vi "test4-MappingRelationshipByLocalRegistration.vi"(8 "error in (no error)":errorcluster, 11 "TestCase in":refnum<class "testcase-CSMStatusStateRegisterUnregister.lvclass">) -> (0 "error out":errorcluster, 3 "TestCase out":refnum<class "testcase-CSMStatusStateRegisterUnregister.lvclass">)   [LabVIEW 2017, in "testcase-CSMStatusStateRegisterUnregister.lvclass"]
uses:
  testcase-CSMStatusStateRegisterUnregister.lvclass
  <vilib>/addons/_JKI Toolkits/VI Tester/TestCase.llb/TestCase.lvclass
  src/user.lib/_NEVSTOP/Communicable State Machine(CSM)/Communicable State Machine.lvlib
  C:/Program Files (x86)/National Instruments/LabVIEW 2017/vi.lib/addons/_JKI Toolkits/VI Tester/TestCase.llb/TestCase.lvclass
panel:
  out "Entries After Removal":T1(array[cluster])
  out "Error Array 2":errorcluster[](array[cluster])
  out "Rules 3":T1(array[cluster])
  out "Status In Registry 3":string[](array[string])
  out "Rules 4":T1(array[cluster])
  out "Status In Registry 4":string[](array[string])
  out "Loop Count 2":i32
  out "Loop Count":i32
  out "Error Array":errorcluster[](array[cluster])
  out "Rules 2":T1(array[cluster])
  out "Status In Registry 2":string[](array[string])
  out "Status In Registry 1":string[](array[string])
  out "Rules 1":T1(array[cluster])
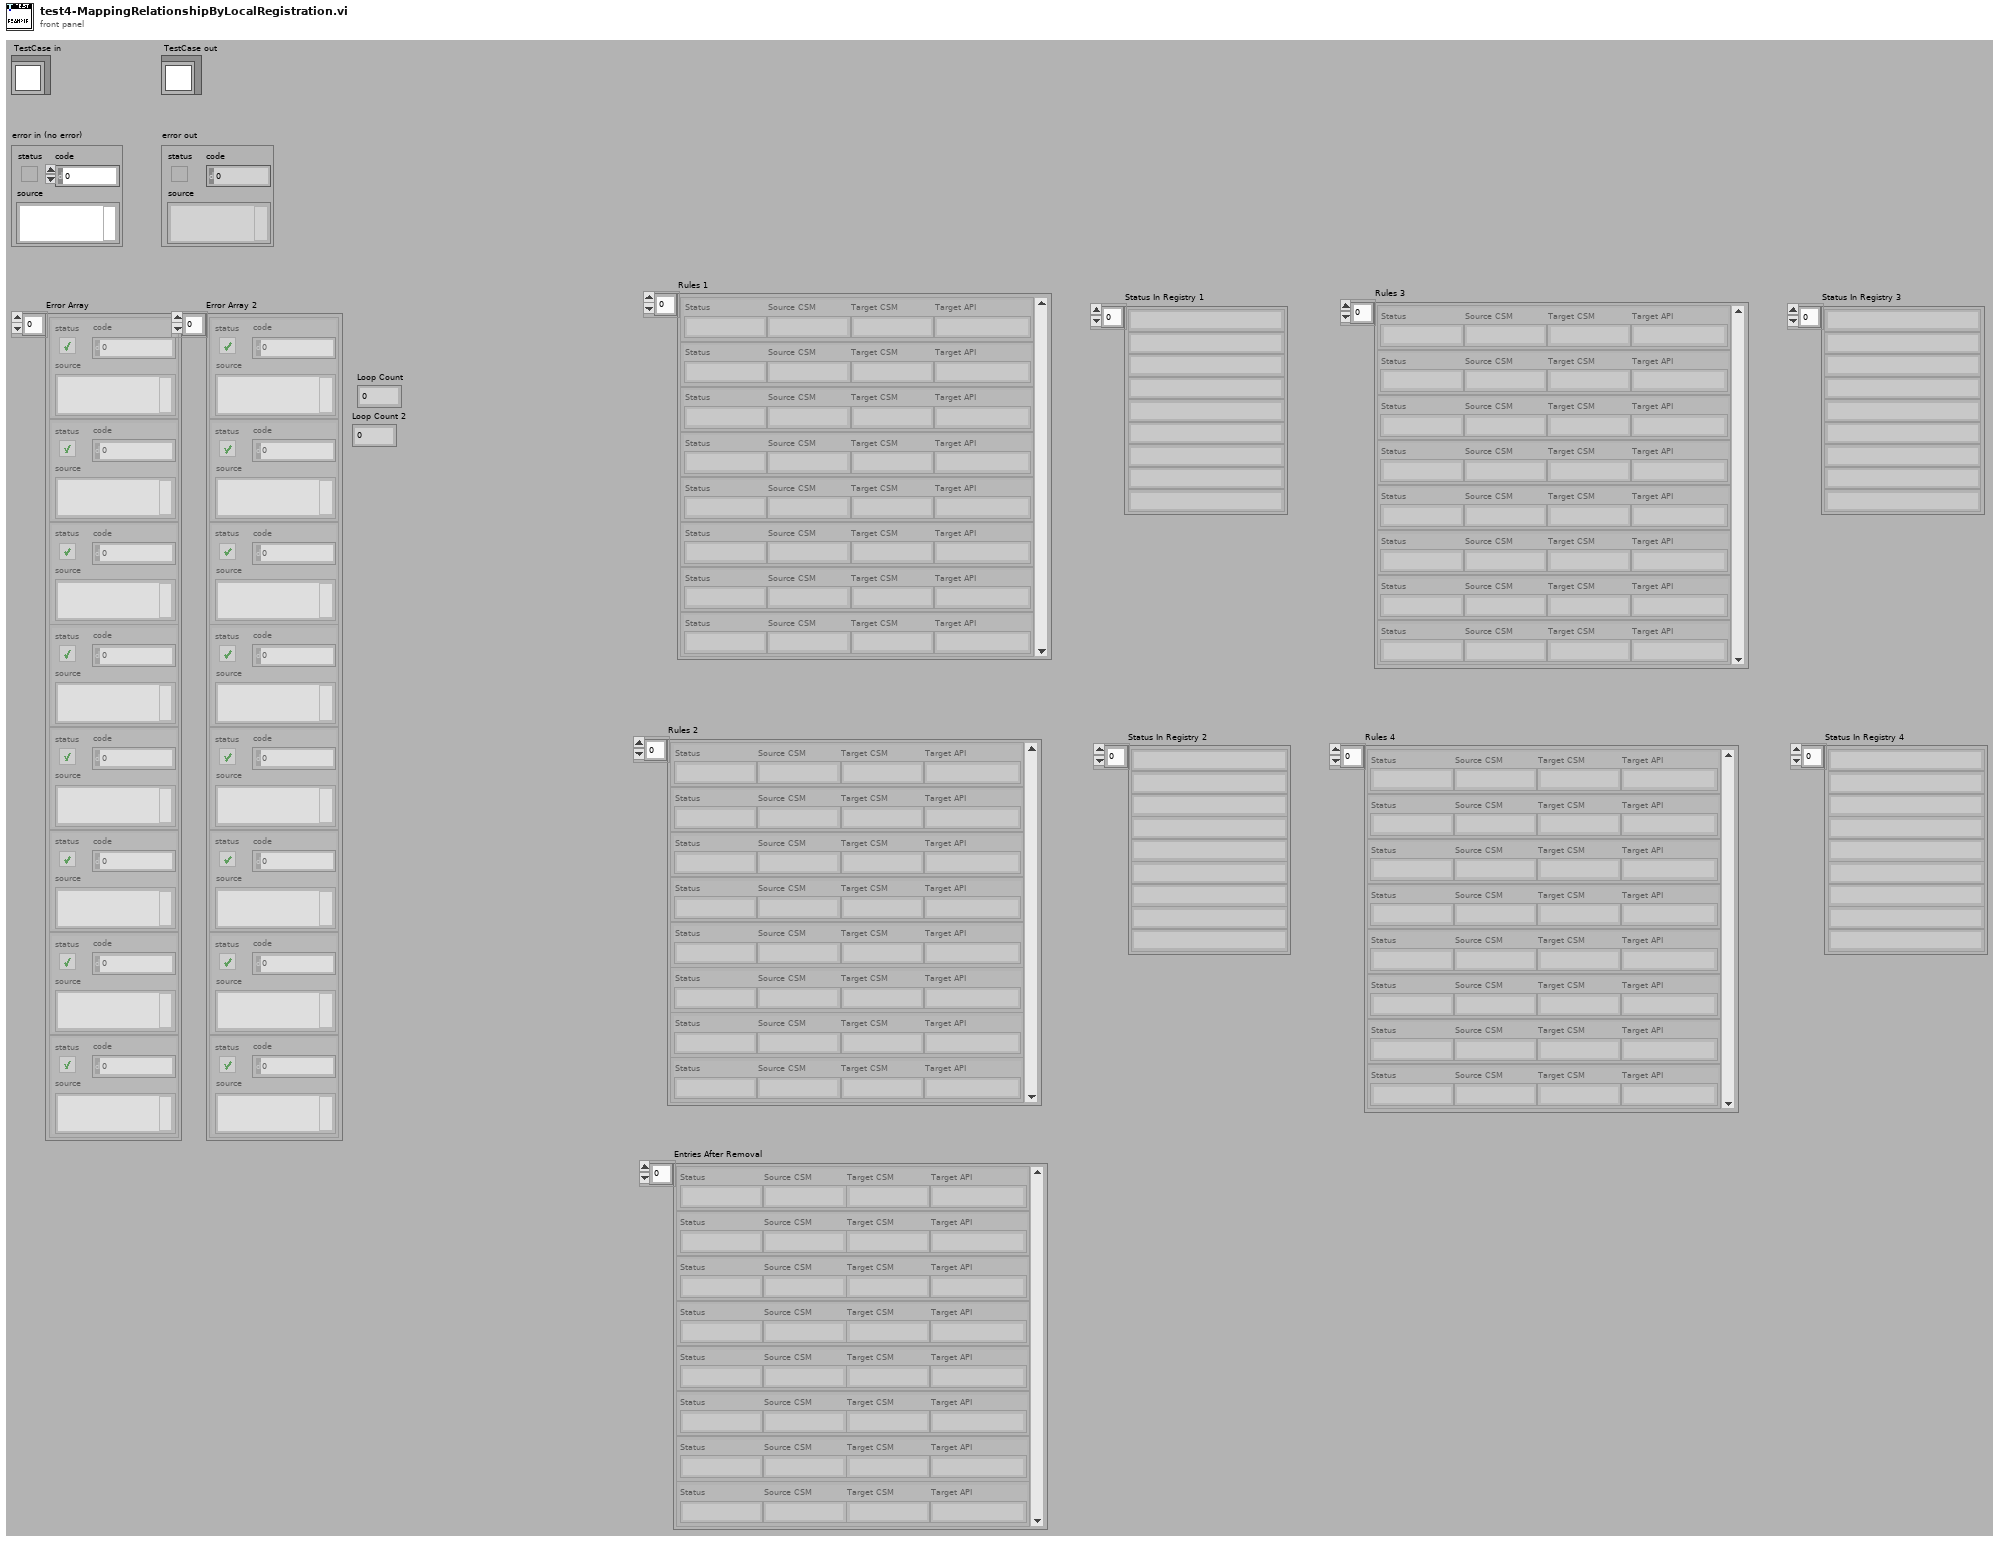
[diagram p1: front panel]
types:
  T1 = cluster{"Status":string, "Source CSM":string, "Target CSM":string, "Target API":string}[]
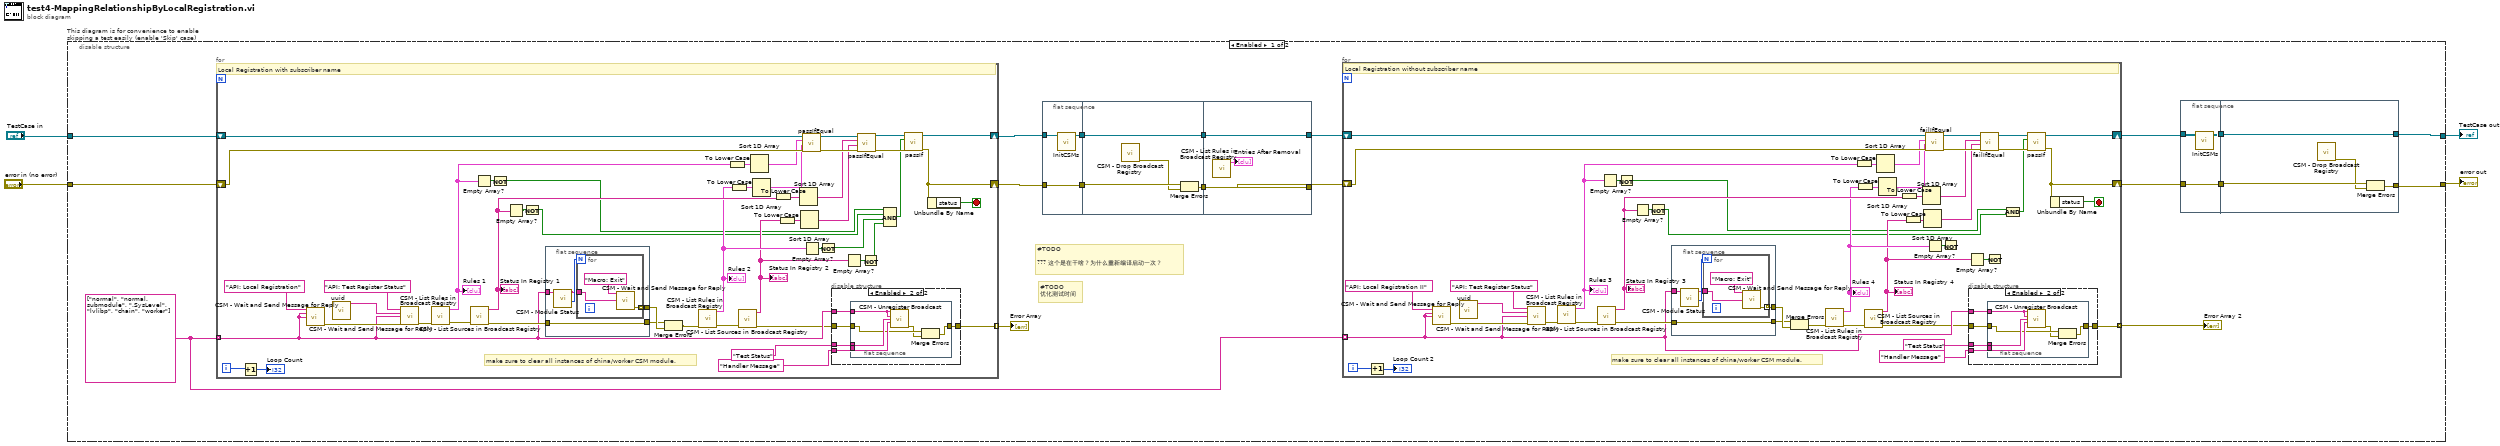
[diagram p0: block diagram]
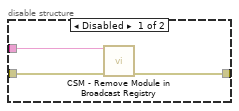
[diagram p2: hidden frame]
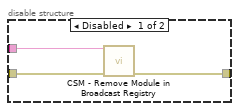
[diagram p3: hidden frame]
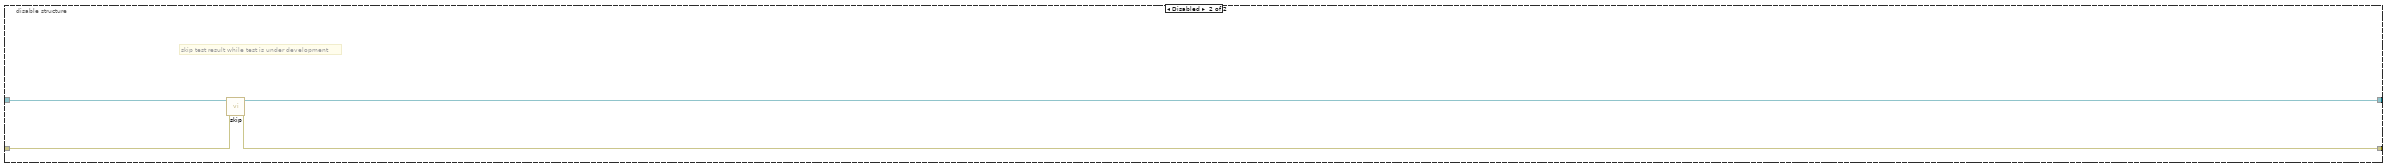
[diagram p4: hidden frame]
diagram:
  n1 = disable-structure "This diagram is for convenience to enable skipping a test easily (enable 'Skip' case)" shown="Enabled" {
    disable-tunnel: "TestCase in" -> [w23 w182]
    disable-tunnel: [w20 w180] -> w1
    disable-tunnel: [w13 w181] -> w3
    disable-tunnel: "error in (no error)" -> [w17 w179]
    frame Enabled {
      w18 = string[] ["normal", "normal.submodule", ".SysLevel", "lvlibp", "chain", "worker"]
      # "#TODO \n优化测试时间"
      # "#TODO \n\n??? 这个是在干啥？为什么重新编译启动一次？"
      n2 = for {
        tunnel: w18 -> [w112] mode=indexing
        shift-right: [w117] -> w10
        shift-left: w23 -> [w149]
        shift-right: [w115] -> w9
        shift-left: w17 -> [w148]
        tunnel: [w113] -> w22 mode=indexing
        i -> [w134]
        stop <- w147 stop-if-true
        # "make sure to clear all instances of china/worker CSM module."
        # "Local Registration with subscriber name"
        n3 = Increment(x=w134) -> (x+1=→"Loop Count":i32)
        n4 = call "CSM - Wait and Send Message for Reply.vi"("State"="API: Local Registration", "Arguments (\"\")"=w112, "Target Module"=w112) -> ("error out"=w155:errorcluster)  [unwired: 10 in, 2 out]
        n5 = call "uuid.vi"() -> ("UUID"=w153:string)  [unwired: 11 in]
        n6 = call "CSM - Wait and Send Message for Reply.vi"("State"="API: Test Register Status", "Arguments (\"\")"=w153, "Target Module"=w112, "Error In (No Error)"=w155) -> ("error out"=w152:errorcluster)  [unwired: 9 in, 2 out]
        n7 = call "CSM - List Rules in Broadcast Registry.vi"("error in (no error)"=w152) -> ("error out"=w146:errorcluster, "Rule Entries"=w130:T1)  [unwired: 9 in]
        "Rules 1" <- w130
        n8 = call "CSM - List Sources in Broadcast Registry.vi"("error in (no error)"=w146) -> ("error out"=w132:errorcluster, "Broadcast Names"=w127:string[])  [unwired: 9 in]
        "Status In Registry 1" <- w127
        n9 = Empty Array?(array=w130) -> (empty?=w129:bool)
        n10 = Not(x=w129) -> (.not. x?=w122:bool)
        n11 = Empty Array?(array=w127) -> (empty?=w128:bool)
        n12 = Not(x=w128) -> (.not. x?=w121:bool)
        n13 = flat-sequence {
          tunnel: [w175] -> w151
          tunnel: w112 -> [w173]
          tunnel: [w172] -> w131
          tunnel: w132 -> [w172]
          frame #0 {
            n14 = call "CSM - Module Status.vi"("CSM Name"=w173) -> ("#Nodes"=w174:i32, "CSM Name (Dup)"=w171:string)  [unwired: 6 in, 3 out]
            n15 = for {
              N: w174 -> [_]
              tunnel: [w177] -> w175 mode=indexing
              tunnel: w171 -> [w176]
              n16 = call "CSM - Wait and Send Message for Reply.vi"("State"="Macro: Exit", "Target Module"=w176) -> ("error out"=w177:errorcluster)  [unwired: 11 in, 2 out]
            }
          }
        }
        n17 = Merge Errors(w131, w151) -> (w150:errorcluster)
        n18 = call "CSM - List Rules in Broadcast Registry.vi"("error in (no error)"=w150) -> ("error out"=w145:errorcluster, "Rule Entries"=w125:T1)  [unwired: 9 in]
        "Rules 2" <- w125
        n19 = To Lower Case(string=w130) -> (all lower case string=w144:T1)
        n20 = To Lower Case(string=w125) -> (all lower case string=w143:T1)
        n21 = call "CSM - List Sources in Broadcast Registry.vi"("error in (no error)"=w145) -> ("error out"=w111:errorcluster, "Broadcast Names"=w123:string[])  [unwired: 9 in]
        "Status In Registry 2" <- w123
        n22 = Sort 1D Array(array=w144) -> (sorted array=w142:T1)
        n23 = Sort 1D Array(array=w143) -> (sorted array=w141:T1)
        n24 = To Lower Case(string=w127) -> (all lower case string=w138:string[])
        n25 = To Lower Case(string=w123) -> (all lower case string=w137:string[])
        n26 = Sort 1D Array(array=w138) -> (sorted array=w136:string[])
        n27 = Sort 1D Array(array=w137) -> (sorted array=w135:string[])
        n28 = call-dynamic "passIfEqual.vi"("error in (no error)"=w148, "y"=w141, "x"=w142, "TestCase in"=w149) -> ("error out"=w139:errorcluster, "TestCase out"=w140:refnum<class "testcase-CSMStatusStateRegisterUnregister.lvclass">)  [unwired: 6 in]
        n29 = Empty Array?(array=w125) -> (empty?=w126:bool)
        n30 = Not(x=w126) -> (.not. x?=w120:bool)
        n31 = disable-structure shown="Enabled" {
          disable-tunnel: w111 -> [w159 w161]
          disable-tunnel: [w158 w160] -> w113
          disable-tunnel: w112 -> [w157 w162]
          disable-tunnel: "Test Status" ("Status") -> [_ w164]
          disable-tunnel: "Handler Message" ("Response Message (If \"\", Same as Source Message)") -> [_ w163]
          frame Disabled {
            n32 = call "CSM - Remove Module in Broadcast Registry.vi"("CSM Name"=w157, "Error In"=w159) -> ("error out"=w158:errorcluster)  [unwired: 12 in, 1 out]
          }
          frame Enabled {
            n33 = flat-sequence {
              tunnel: w164 -> [w170]
              tunnel: w163 -> [w169]
              tunnel: w162 -> [w168]
              tunnel: w161 -> [w167]
              tunnel: [w165] -> w160
              frame #0 {
                n34 = call "CSM - Unregister Broadcast.vi"("CSM Name"=w168, "Source CSM Name (* as Default)"=w168, "Trigger"=w170, "API (\"*\" as Default)"=w169) -> ("error out"=w166:errorcluster)  [unwired: 10 in, 1 out]
                n35 = Merge Errors(w167, w166) -> (w165:errorcluster)
              }
            }
          }
        }
        n36 = Empty Array?(array=w123) -> (empty?=w124:bool)
        n37 = call-dynamic "passIfEqual.vi"("error in (no error)"=w139, "y"=w135, "x"=w136, "TestCase in"=w140) -> ("error out"=w116:errorcluster, "TestCase out"=w118:refnum<class "testcase-CSMStatusStateRegisterUnregister.lvclass">)  [unwired: 6 in]
        n38 = Not(x=w124) -> (.not. x?=w119:bool)
        n39 = Compound Arithmetic op=AND(w122, w121, w120, w119) -> (w114:bool)
        n40 = call-dynamic "passIf.vi"("error in (no error)"=w116, "pass"=w114, "TestCase in"=w118) -> ("error out"=w115:errorcluster, "TestCase out"=w117:refnum<class "testcase-CSMStatusStateRegisterUnregister.lvclass">)  [unwired: 7 in]
        n41 = Unbundle By Name(w115) -> ("status"=w147:bool)
      }
      "Error Array" <- w22
      n42 = flat-sequence {
        tunnel: w10 -> [w26]
        tunnel: [w25] -> w12
        tunnel: [w24] -> w11
        tunnel: w9 -> [w24]
        tunnel: w12 -> [w30]
        tunnel: w11 -> [w29]
        tunnel: [w30] -> w6
        tunnel: [w28] -> w5
        tunnel: [w32] -> w7
        tunnel: [w33] -> w8
        tunnel: w6 -> [w33]
        tunnel: w5 -> [w32]
        frame #0 {
          n43 = call "InitCSMs.vi"("testcase-CSMStatus in"=w26) -> ("testcase-CSMStatus out"=w25:refnum<class "testcase-CSMStatusStateRegisterUnregister.lvclass">)  [unwired: 9 in, 1 out]
        }
        frame #1 {
          n44 = call "CSM - Drop Broadcast Registry.vi"() -> ("error out"=w27:errorcluster)  [unwired: 15 in]
          n45 = Merge Errors(w29, w27) -> (w28:errorcluster)
        }
        frame #2 {
          n46 = call "CSM - List Rules in Broadcast Registry.vi"() -> ("Rule Entries"=→"Entries After Removal":T1)  [unwired: 10 in, 1 out]
        }
      }
      n47 = for {
        tunnel: w18 -> [w44] mode=indexing
        shift-right: [w49] -> w21
        shift-left: w8 -> [w79]
        shift-right: [w47] -> w14
        shift-left: w7 -> [w78]
        tunnel: [w45] -> w19 mode=indexing
        i -> [w64]
        stop <- w77 stop-if-true
        # "make sure to clear all instances of china/worker CSM module."
        # "Local Registration without subscriber name"
        n48 = Increment(x=w64) -> (x+1=→"Loop Count 2":i32)
        n49 = call "CSM - Wait and Send Message for Reply.vi"("State"="API: Local Registration II", "Arguments (\"\")"=w44, "Target Module"=w44) -> ("error out"=w85:errorcluster)  [unwired: 10 in, 2 out]
        n50 = call "uuid.vi"() -> ("UUID"=w83:string)  [unwired: 11 in]
        n51 = call "CSM - Wait and Send Message for Reply.vi"("State"="API: Test Register Status", "Arguments (\"\")"=w83, "Target Module"=w44, "Error In (No Error)"=w85) -> ("error out"=w82:errorcluster)  [unwired: 9 in, 2 out]
        n52 = call "CSM - List Rules in Broadcast Registry.vi"("error in (no error)"=w82) -> ("error out"=w76:errorcluster, "Rule Entries"=w60:T1)  [unwired: 9 in]
        "Rules 3" <- w60
        n53 = call "CSM - List Sources in Broadcast Registry.vi"("error in (no error)"=w76) -> ("error out"=w62:errorcluster, "Broadcast Names"=w57:string[])  [unwired: 9 in]
        "Status In Registry 3" <- w57
        n54 = Empty Array?(array=w60) -> (empty?=w59:bool)
        n55 = Not(x=w59) -> (.not. x?=w52:bool)
        n56 = Empty Array?(array=w57) -> (empty?=w58:bool)
        n57 = Not(x=w58) -> (.not. x?=w51:bool)
        n58 = flat-sequence {
          tunnel: [w105] -> w81
          tunnel: w44 -> [w103]
          tunnel: [w102] -> w61
          tunnel: w62 -> [w102]
          frame #0 {
            n59 = call "CSM - Module Status.vi"("CSM Name"=w103) -> ("#Nodes"=w104:i32, "CSM Name (Dup)"=w101:string)  [unwired: 6 in, 3 out]
            n60 = for {
              N: w104 -> [_]
              tunnel: [w107] -> w105 mode=indexing
              tunnel: w101 -> [w106]
              n61 = call "CSM - Wait and Send Message for Reply.vi"("State"="Macro: Exit", "Target Module"=w106) -> ("error out"=w107:errorcluster)  [unwired: 11 in, 2 out]
            }
          }
        }
        n62 = Merge Errors(w61, w81) -> (w80:errorcluster)
        n63 = call "CSM - List Rules in Broadcast Registry.vi"("error in (no error)"=w80) -> ("error out"=w75:errorcluster, "Rule Entries"=w55:T1)  [unwired: 9 in]
        "Rules 4" <- w55
        n64 = To Lower Case(string=w60) -> (all lower case string=w74:T1)
        n65 = To Lower Case(string=w55) -> (all lower case string=w73:T1)
        n66 = call "CSM - List Sources in Broadcast Registry.vi"("error in (no error)"=w75) -> ("error out"=w43:errorcluster, "Broadcast Names"=w53:string[])  [unwired: 9 in]
        "Status In Registry 4" <- w53
        n67 = Sort 1D Array(array=w74) -> (sorted array=w72:T1)
        n68 = Sort 1D Array(array=w73) -> (sorted array=w71:T1)
        n69 = To Lower Case(string=w57) -> (all lower case string=w68:string[])
        n70 = To Lower Case(string=w53) -> (all lower case string=w67:string[])
        n71 = Sort 1D Array(array=w68) -> (sorted array=w66:string[])
        n72 = Sort 1D Array(array=w67) -> (sorted array=w65:string[])
        n73 = call-dynamic "failIfEqual.vi"("error in (no error)"=w78, "y"=w71, "x"=w72, "TestCase in"=w79) -> ("error out"=w69:errorcluster, "TestCase out"=w70:refnum<class "testcase-CSMStatusStateRegisterUnregister.lvclass">)  [unwired: 6 in]
        n74 = Empty Array?(array=w55) -> (empty?=w56:bool)
        n75 = Not(x=w56) -> ()  [unwired: 1 out]
        n76 = Empty Array?(array=w53) -> (empty?=w54:bool)
        n77 = disable-structure shown="Enabled" {
          disable-tunnel: w43 -> [w89 w91]
          disable-tunnel: [w88 w90] -> w45
          disable-tunnel: w44 -> [w87 w92]
          disable-tunnel: "Test Status" ("Status") -> [_ w94]
          disable-tunnel: "Handler Message" ("Response Message (If \"\", Same as Source Message)") -> [_ w93]
          frame Disabled {
            n78 = call "CSM - Remove Module in Broadcast Registry.vi"("CSM Name"=w87, "Error In"=w89) -> ("error out"=w88:errorcluster)  [unwired: 12 in, 1 out]
          }
          frame Enabled {
            n79 = flat-sequence {
              tunnel: w94 -> [w100]
              tunnel: w93 -> [w99]
              tunnel: w92 -> [w98]
              tunnel: w91 -> [w97]
              tunnel: [w95] -> w90
              frame #0 {
                n80 = call "CSM - Unregister Broadcast.vi"("CSM Name"=w98, "Source CSM Name (* as Default)"=w98, "Trigger"=w100, "API (\"*\" as Default)"=w99) -> ("error out"=w96:errorcluster)  [unwired: 10 in, 1 out]
                n81 = Merge Errors(w97, w96) -> (w95:errorcluster)
              }
            }
          }
        }
        n82 = call-dynamic "failIfEqual.vi"("error in (no error)"=w69, "y"=w65, "x"=w66, "TestCase in"=w70) -> ("error out"=w48:errorcluster, "TestCase out"=w50:refnum<class "testcase-CSMStatusStateRegisterUnregister.lvclass">)  [unwired: 6 in]
        n83 = Not(x=w54) -> ()  [unwired: 1 out]
        n84 = Compound Arithmetic op=AND(w52, w51) -> (w46:bool)
        n85 = call-dynamic "passIf.vi"("error in (no error)"=w48, "pass"=w46, "TestCase in"=w50) -> ("error out"=w47:errorcluster, "TestCase out"=w49:refnum<class "testcase-CSMStatusStateRegisterUnregister.lvclass">)  [unwired: 7 in]
        n86 = Unbundle By Name(w47) -> ("status"=w77:bool)
      }
      "Error Array 2" <- w19
      n87 = flat-sequence {
        tunnel: w21 -> [w36]
        tunnel: [w35] -> w16
        tunnel: [w34] -> w15
        tunnel: w14 -> [w34]
        tunnel: [w40] -> w20
        tunnel: w16 -> [w40]
        tunnel: w15 -> [w39]
        tunnel: [w38] -> w13
        frame #0 {
          n88 = call "InitCSMs.vi"("testcase-CSMStatus in"=w36) -> ("testcase-CSMStatus out"=w35:refnum<class "testcase-CSMStatusStateRegisterUnregister.lvclass">)  [unwired: 9 in, 1 out]
        }
        frame #1 {
          n89 = call "CSM - Drop Broadcast Registry.vi"() -> ("error out"=w37:errorcluster)  [unwired: 15 in]
          n90 = Merge Errors(w39, w37) -> (w38:errorcluster)
        }
      }
    }
    frame Disabled {
      # "skip test result while test is under development"
      n91 = call <vilib>:"skip.vi"("error in (no error)"=w179, "TestCase in"=w182) -> ("error out"=w181:errorcluster, "TestCase out"=w180:refnum<class "testcase-CSMStatusStateRegisterUnregister.lvclass">)  [unwired: 8 in]
    }
  }
  "error out" <- w3
  "TestCase out" <- w1
